vi "Add Next Item Number.vi"(0 "Array in":u8[](array[numeric])) -> (1 "Array out":u8[](array[numeric]), 2 "Added":u8)   [LabVIEW 2018]
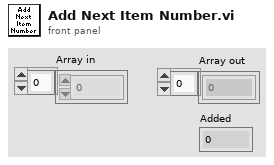
[diagram p1: front panel]
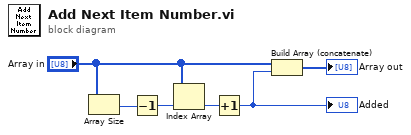
[diagram p0: block diagram]
diagram:
  n1 = Array Size(array="Array in") -> (size(s)=w3:i32)
  n2 = Decrement(x=w3) -> (x-1=w4:i32)
  n3 = Index Array(array="Array in", index=w4) -> (element=w2:u8)
  n4 = Increment(x=w2) -> (x+1=w1:u8)
  "Added" <- w1
  n5 = Build Array (concatenate)("Array in", w1) -> (→"Array out":u8[])
